vi "Log Prompt Async.vi"(7 "VolatusAPI":refnum<class "VolatusAPI.lvclass">, 9 "Target (All)":string, 10 "Log Group (All)":T1, 11 "LoggingControl in":refnum<class "GroupLoggingControl.lvclass">) -> ()   [LabVIEW 2020, in "VolatusGUIElements.lvlib" / "GroupLoggingControl.lvclass"]
uses:
  GroupLoggingControl.lvclass
  Volatus/VolatusAPI/VolatusAPI.lvclass
  Log Group.ctl
  Log Group Status.ctl
  Command Info.ctl
  GroupLoggingControl.lvclass/GroupLoggingControl.ctl
  lv-cdm/CDM-Config/ISO8601 Config.ctl
  lv-cdm/CDM-Config/Format.ctl
  lv-cdm/CDM-Config/Precision.ctl
  lv-cdm/CDM-Config/Timezone.ctl
  messages/StartLog/Data.ctl
  Prompt Result.ctl
  Prompt Action.ctl
  messages/StartLog/Class/Msg.lvclass/Msg.ctl
  Volatus/VolatusAPI/VolatusAPI.lvclass/VolatusAPI.ctl
  messages/StartLog/Class/Msg.lvclass
  C:/dev/lv20CE/relink/lv-protoc/LV-Proto/Message/Message.lvclass
  lv-cdm/CDM-Config/ISO-8601 Format Strings.vi
  lv-vecto/Vecto/TCPMessageService/Send Message.vi
  <vilib>/Utility/error.llb/Error Cluster From Error Code.vi
  lv-protoc/LV-Proto/Message/Message.lvclass
  lv-cdm/CDM-Config/CDM-Config.lvlib
  messages/StartLog/StartLog.lvlib
  C:/dev/lv20CE/relink/lv-volatus/messages/StartLog/Class/Msg.lvclass
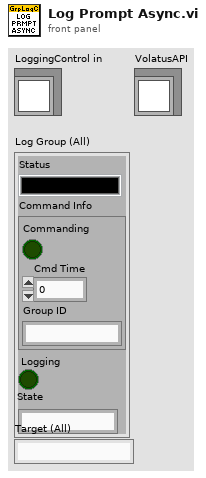
[diagram p1: front panel]
types:
  T1 = typedef "VolatusGUIElements.lvlib/GroupLoggingControl.lvclass/Log Group.ctl" = cluster{"Status":T2, "Command Info":T3, "Logging":bool, "State":string}
  T2 = typedef "VolatusGUIElements.lvlib/GroupLoggingControl.lvclass/Log Group Status.ctl" = cluster{"Group":string, "Group Color":u32, "Button":bool}
  T3 = typedef "VolatusGUIElements.lvlib/GroupLoggingControl.lvclass/Command Info.ctl" = cluster{"Commanding":bool, "Cmd Time":dbl, "Group ID":string}
  T4 = typedef "VolatusGUIElements.lvlib/GroupLoggingControl.lvclass/Status.ctl" = cluster{"Groups":T1[], "Targets":T5[]}
  T5 = typedef "VolatusGUIElements.lvlib/GroupLoggingControl.lvclass/Target Info.ctl" = cluster{"Node":string, "Node Color":u32, "Groups":T1[]}
  T6 = typedef "VolatusGUIElements.lvlib/GroupLoggingControl.lvclass/Prompt Action.ctl" = enum16{"Cancelled", "Started"}
  T7 = typedef "VolatusGUIElements.lvlib/GroupLoggingControl.lvclass/Prompt Result.ctl" = cluster{"Action":T6, "Series":string, "Timestamp":string, "Target (All)":string, "Group (All)":string}
  T8 = typedef "StartLog.lvlib/Data.ctl" = cluster{"series":string, "timestamp":string, "started_by":string, "groups":string[]}
  T9 = typedef "CDM-Config.lvlib/ISO8601 Config.ctl" = cluster{"Format":T10, "Precision":T11, "Timezone":T12}
  T10 = typedef "CDM-Config.lvlib/Format.ctl" = enum16{"Extended", "Basic"}
  T11 = typedef "CDM-Config.lvlib/Precision.ctl" = enum16{"Millisecond", "Second", "Minute", "Hour", "Day"}
  T12 = typedef "CDM-Config.lvlib/Timezone.ctl" = enum16{"UTC", "Local"}
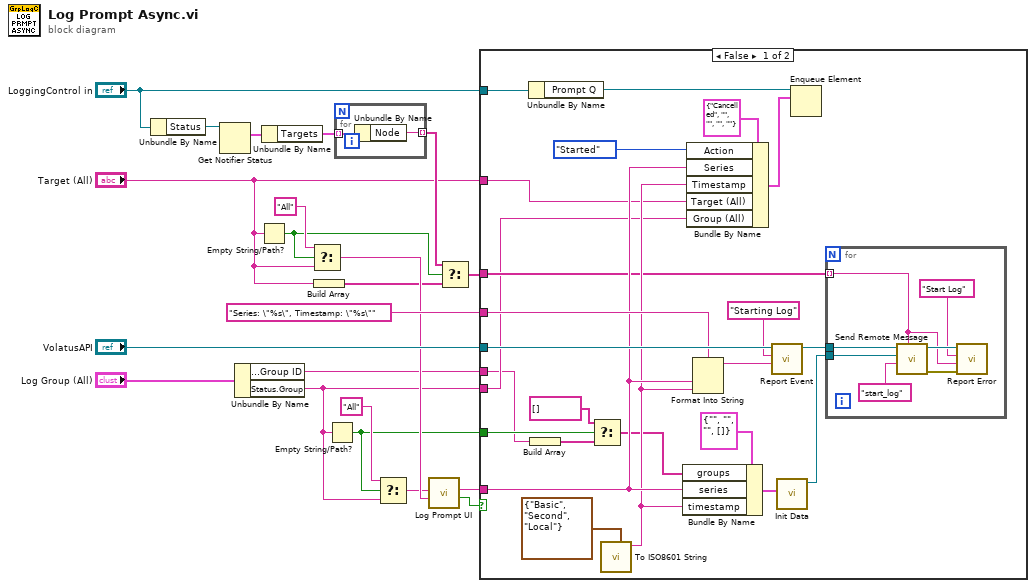
[diagram p0: block diagram]
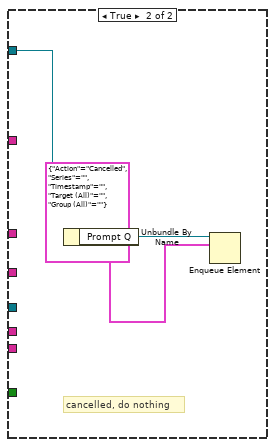
[diagram p2: hidden frame]
diagram:
  n1 = Unbundle By Name("LoggingControl in") -> ("Status"=w2:refnum<notifier>)
  n2 = Get Notifier Status(notifier=w2) -> (current notification=w1:T4)  [unwired: 1 in, 4 out]
  n3 = Unbundle By Name("Log Group (All)") -> ("Command Info.Group ID"=w4:string, "Status.Group"=w6:string)
  n4 = Empty String/Path?(string/path="Target (All)") -> (empty?=w11:bool)
  n5 = Unbundle By Name(w1) -> ("Targets"=w12:T5[])
  n6 = Select(t="All", s=w11, f="Target (All)") -> (s? t:f=w17:string)
  n7 = Build Array("Target (All)") -> (w9:string[])
  n8 = Empty String/Path?(string/path=w6) -> (empty?=w5:bool)
  n9 = for {
    tunnel: w12 -> [w23] mode=indexing
    tunnel: [w22] -> w10 mode=indexing
    n10 = Unbundle By Name(w23) -> ("Node"=w22:string)
  }
  n11 = Select(t="All", s=w5, f=w6) -> (s? t:f=w15:string)
  n12 = call "Log Prompt UI.vi"("Target Prompt"=w17, "Group Prompt"=w15) -> ("Cancelled"=w21:bool, "Series"=w20:string)  [unwired: 8 in]
  n13 = Select(t=w10, s=w11, f=w9) -> (s? t:f=w8:string[])
  n14 = case shown="False" w21 {
    tunnel: w20 -> [w33 _]
    tunnel: "LoggingControl in" -> [w44 w57]
    tunnel: "VolatusAPI" -> [w43 _]
    tunnel: "Series: \"%s\", Timestamp: \"%s\"" -> [w34 _]
    tunnel: w8 -> [w31 _]
    tunnel: "Target (All)" -> [w30 _]
    tunnel: w6 -> [w29 _]
    tunnel: w5 -> [w28 _]
    tunnel: w4 -> [w24 _]
    frame False {
      n15 = Unbundle By Name(w44) -> ("Prompt Q"=w38:refnum<queue>)
      n16 = Build Array(w24) -> (w27:string[])
      n17 = Select(t=string[] [], s=w28, f=w27) -> (s? t:f=w25:string[])
      n18 = call "To ISO8601 String.vi"("Format Config"=T9 {"Format"=enum."Basic", "Precision"=enum."Second", "Timezone"=enum."Local"}) -> ("ISO 8601"=w32:string)  [unwired: 10 in]
      n19 = Bundle By Name(cluster=T8 {"series"="", "timestamp"="", "started_by"="", "groups"=[]} ("Data"), "groups"=w25, "series"=w33, "timestamp"=w32) -> (w45:T8)
      n20 = Bundle By Name(cluster=T7 {"Action"=enum."Cancelled", "Series"="", "Timestamp"="", "Target (All)"="", "Group (All)"=""} ("Prompt Result"), "Action"=Prompt_Action."Started", "Series"=w33, "Timestamp"=w32, "Target (All)"=w30, "Group (All)"=w29) -> (w41:T7)
      n21 = Format Into String(format string=w34, w33, w32) -> (resulting string=w35:string)  [unwired: 2 in, 1 out]
      n22 = call "Report Event.vi"("Message"=w35, "Context"="Starting Log", "VolatusAPI in"=w43) -> ("VolatusAPI out"=w37:refnum<class "VolatusAPI.lvclass">)  [unwired: 7 in, 1 out]
      n23 = call "Init Data.vi"("Data"=w45) -> ("Msg out"=w42:refnum<class "Msg.lvclass">)  [unwired: 10 in]
      n24 = Enqueue Element(queue=w38, element=w41) -> ()  [unwired: 2 in, 3 out]
      n25 = for {
        tunnel: w37 -> [w54]
        tunnel: w42 -> [w53]
        tunnel: w31 -> [w48] mode=indexing
        n26 = call "Send Remote Message.vi"("Target Name"=w48, "Message Type"="start_log", "Message"=w53, "VolatusAPI in"=w54) -> ("error out"=w49:errorcluster, "VolatusAPI out"=w51:refnum<class "VolatusAPI.lvclass">)  [unwired: 6 in]
        n27 = call "Report Error.vi"("error in (no error)"=w49, "Message"=w48, "Context"="Start Log", "VolatusAPI in"=w51) -> ()  [unwired: 6 in, 2 out]
      }
    }
    frame True {
      # "cancelled, do nothing"
      n28 = Unbundle By Name(w57) -> ("Prompt Q"=w56:refnum<queue>)
      n29 = Enqueue Element(queue=w56, element=T7 {"Action"=enum."Cancelled", "Series"="", "Timestamp"="", "Target (All)"="", "Group (All)"=""}) -> ()  [unwired: 2 in, 3 out]
    }
  }
